vi "Set File Conflict Operation.vi"(8 "error in (no error)":errorcluster, 10 "File Conflict Operation":T1, 11 "Log File Specification in":refnum<class "Log File Specification.lvclass">) -> (0 "error out":errorcluster, 3 "Log File Specification out":refnum<class "Log File Specification.lvclass">)   [LabVIEW 2015, in "Log File Specification.lvclass"]
uses:
  Log File Specification.lvclass
  File Conflict Operation.ctl
  Log File Specification.lvclass/Log File Specification.ctl
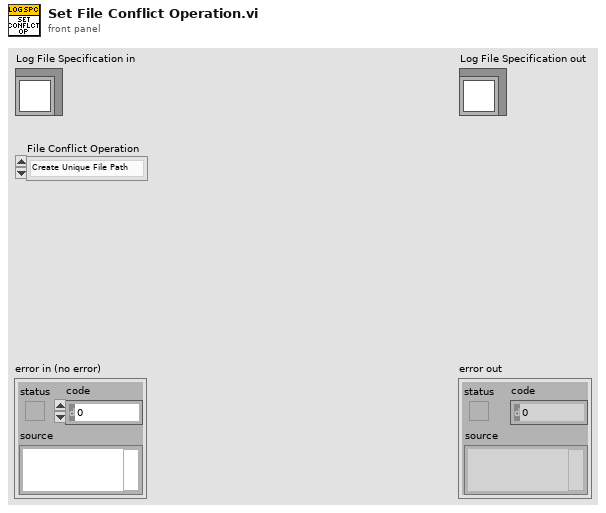
[diagram p1: front panel]
types:
  T1 = typedef "Log File Specification.lvclass/File Conflict Operation.ctl" = enum16{"Create Unique File Path", "Append to Existing", "Overwrite Existing"}
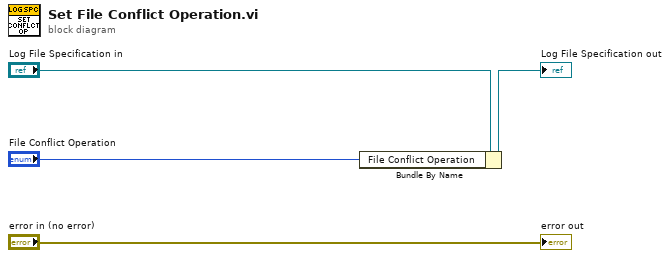
[diagram p0: block diagram]
diagram:
  n1 = Bundle By Name(cluster="Log File Specification in", "File Conflict Operation"="File Conflict Operation") -> (→"Log File Specification out":refnum<class "Log File Specification.lvclass">)
  "error out" <- "error in (no error)"
